vi "labview_read_serial_com_port.vi"() -> ()   [LabVIEW 2018]
uses:
  <vilib>/Instr/_visa.llb/VISA Configure Serial Port (Instr).vi
panel:
  out "Waveform Chart":dbl(graph)
  out "read buffer":string
  out "error out 2":errorcluster
  in  "COM port 2":refnum<visa-resource-name>
  out "error out":errorcluster
  in  "write buffer":string
  in  "COM Port 1":refnum<visa-resource-name>
  in  "stop":bool
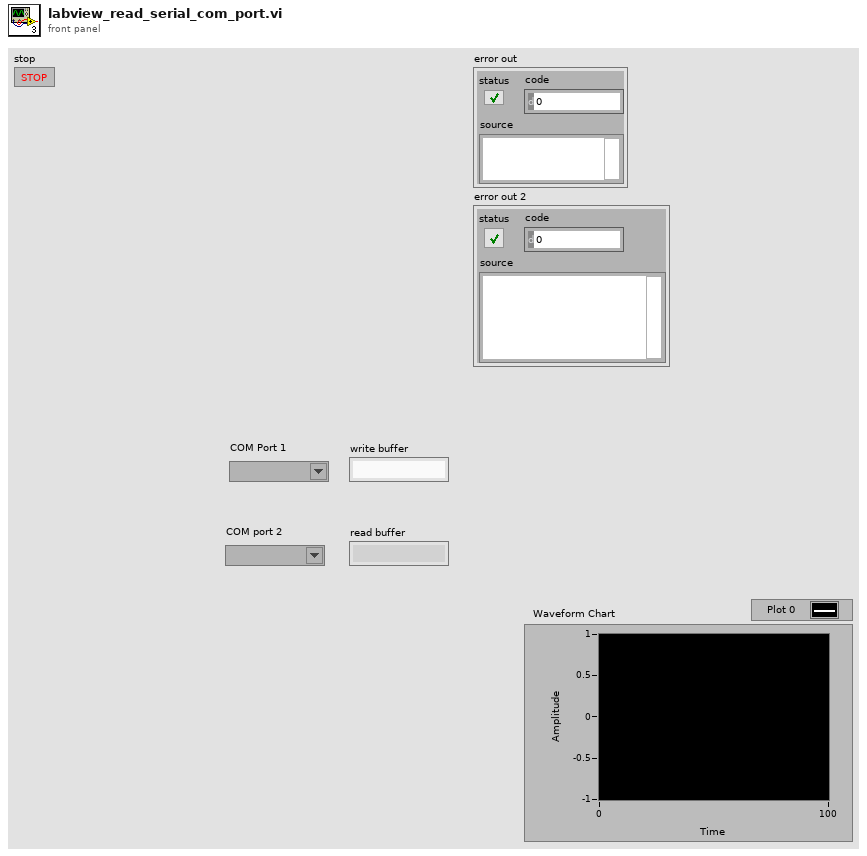
[diagram p1: front panel]
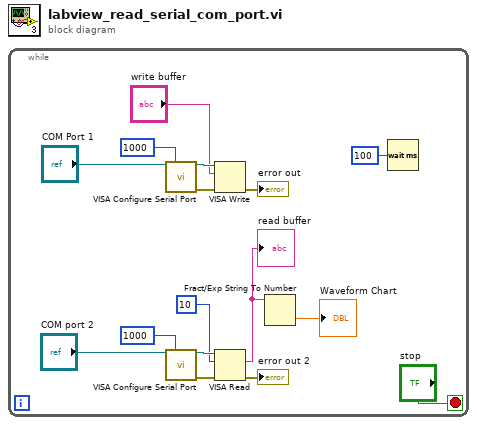
[diagram p0: block diagram]
diagram:
  n1 = while {
    stop <- "stop" stop-if-true
    n2 = call-poly "VISA Configure Serial Port"("VISA resource name"="COM Port 1", "timeout (10sec)"=u32 1000) -> ("VISA resource name out"=w14:refnum<visa-resource-name>, "error out"=w12:errorcluster)  [unwired: 12 in]
    n3 = call-poly "VISA Configure Serial Port"("VISA resource name"="COM port 2", "timeout (10sec)"=u32 1000) -> ("VISA resource name out"=w9:refnum<visa-resource-name>, "error out"=w8:errorcluster)  [unwired: 12 in]
    n4 = VISA Write(VISA resource name=w14, write buffer="write buffer", error in (no error)=w12) -> (error out=→"error out":errorcluster)  [unwired: 2 out]
    n5 = VISA Read(VISA resource name=w9, byte count=u32 10, error in (no error)=w8) -> (read buffer=w2:string, error out=→"error out 2":errorcluster)  [unwired: 2 out]
    "read buffer" <- w2
    n6 = Fract/Exp String To Number(string=w2) -> (number=→"Waveform Chart":dbl)  [unwired: 3 in, 1 out]
    n7 = Wait (ms)(milliseconds to wait=u32 100) -> ()  [unwired: 1 out]
  }
